vi "DSF.Engine.Pointer.Status.Builder.State.New.vi"(8 "error in (no error)":errorcluster, 10 "count (1)":u64=1, 11 "Builder State Pointer type":refnum<class "DSF.Engine.Pointer.Status.Builder.State.lvclass">) -> (0 "error out":errorcluster, 3 "Builder State Pointer":refnum<class "DSF.Engine.Pointer.Status.Builder.State.lvclass">)   [LabVIEW 2017, in "DSF.Engine.lvlib" / "DSF.Engine.Pointer.Status.Builder.State.lvclass"]
uses:
  Pointer/DSF.Engine.Pointer.Status.Builder.State.lvclass
  C:/Git/DSF/dsf core/Built/Windows/Dependencies/Memory Manager.lvlibp/1abvi3w/vi.lib/National Instruments/Memory Manager/Classes/Pointer/Memory.Pointer.lvclass
  Built/Windows/Dependencies/Memory Manager.lvlibp/1abvi3w/vi.lib/National Instruments/Memory Manager/Classes/Pointer/Memory.Pointer.New.1B.vi
  Built/Windows/Dependencies/Memory Manager.lvlibp/1abvi3w/vi.lib/National Instruments/Memory Manager/Classes/Pointer/Memory.Pointer.lvclass
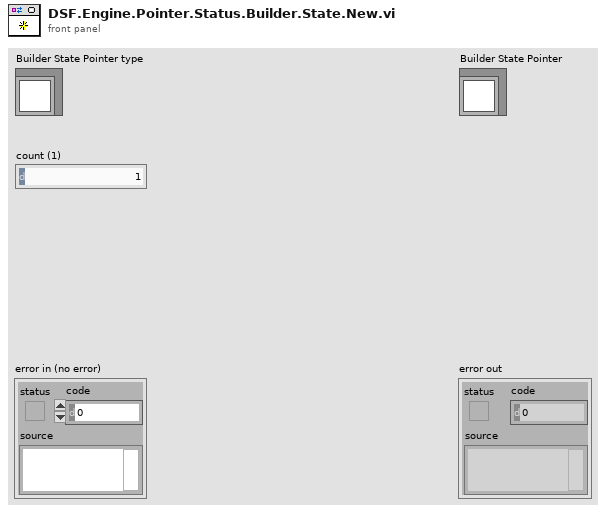
[diagram p1: front panel]
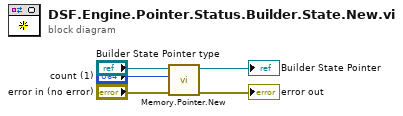
[diagram p0: block diagram]
diagram:
  n1 = call-poly "Memory.Pointer.New.vi"("error in (no error)"="error in (no error)", "count (1)"="count (1)", "Pointer type"="Builder State Pointer type") -> ("error out"=→"error out":errorcluster, "Pointer"=→"Builder State Pointer":refnum<class "DSF.Engine.Pointer.Status.Builder.State.lvclass">)  [unwired: 7 in]
